vi "DisposeCore.vi"(8 "error in (no error)":errorcluster, 11 "BombedWall":refnum<class "BombedWall.lvclass">) -> (0 "error out":errorcluster, 3 "BombedWall":refnum<class "BombedWall.lvclass">)   [LabVIEW 2020, in "BombedWall.lvclass"]
uses:
  BombedWall.lvclass
  Private/TypeDef/privateDataDVR.ctl
  Private/TypeDef/privateData.ctl
  BombedWall.lvclass/BombedWall.ctl
  Wall/Wall.lvclass
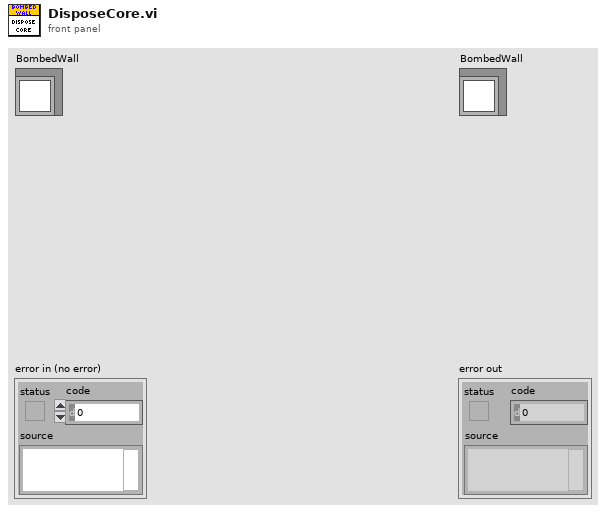
[diagram p1: front panel]
types:
  T1 = typedef "BombedWall.lvclass/privateDataDVR.ctl" = refnum<data-value>
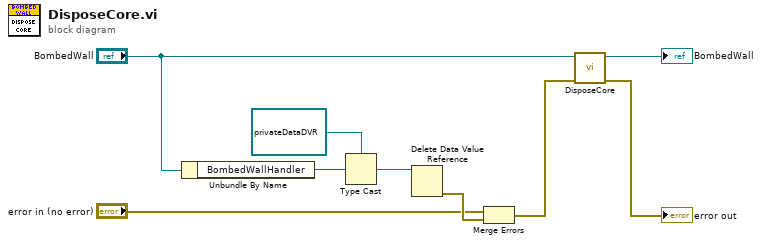
[diagram p0: block diagram]
diagram:
  n1 = Unbundle By Name("BombedWall") -> ("BombedWallHandler"=w8:u32)
  n2 = Type Cast(type=T1 refnum ("privateDataDVR"), x=w8) -> (*(type *) &x=w9:T1)
  n3 = Delete Data Value Reference(data value reference=w9) -> (error out=w7:errorcluster)  [unwired: 1 in, 1 out]
  n4 = Merge Errors("error in (no error)", w7) -> (w2:errorcluster)
  n5 = call-parent "DisposeCore.vi"("error in (no error)"=w2, "Wall"="BombedWall") -> ("error out"=→"error out":errorcluster, "Wall"=→"BombedWall":refnum<class "BombedWall.lvclass">)  [unwired: 8 in]
